vi "Test Sequencer.vi"(7 "Initial Data":T3={"Model Name"=enum."W 501 FLH Std.", "ID"="ID", "Shift"=""}, 8 "Error In":errorcluster, 9 "Initialize":bool, 10 "Inputs":T6) -> (0 "Error Out":errorcluster, 1 "Completed?":bool, 2 "Results":T4, 3 "Results Cluster out":T1, 4 "Graph":dbl[][](array[numeric]), 5 "TS Status":cluster{"Status":string, "Elapsed Time":dbl})   [LabVIEW 2017]
uses:
  controls/All Inputs.ctl
  controls/SACB DI.ctl
  controls/Test Sequencer.ctl
  controls/AC Results.ctl
  controls/Model Name.ctl
  controls/Results Cluster.ctl
  controls/Result Checker.ctl
  GV/Specs.vi
  support/GV/Towerlight GV.vi
panel:
  out "Current State":T5
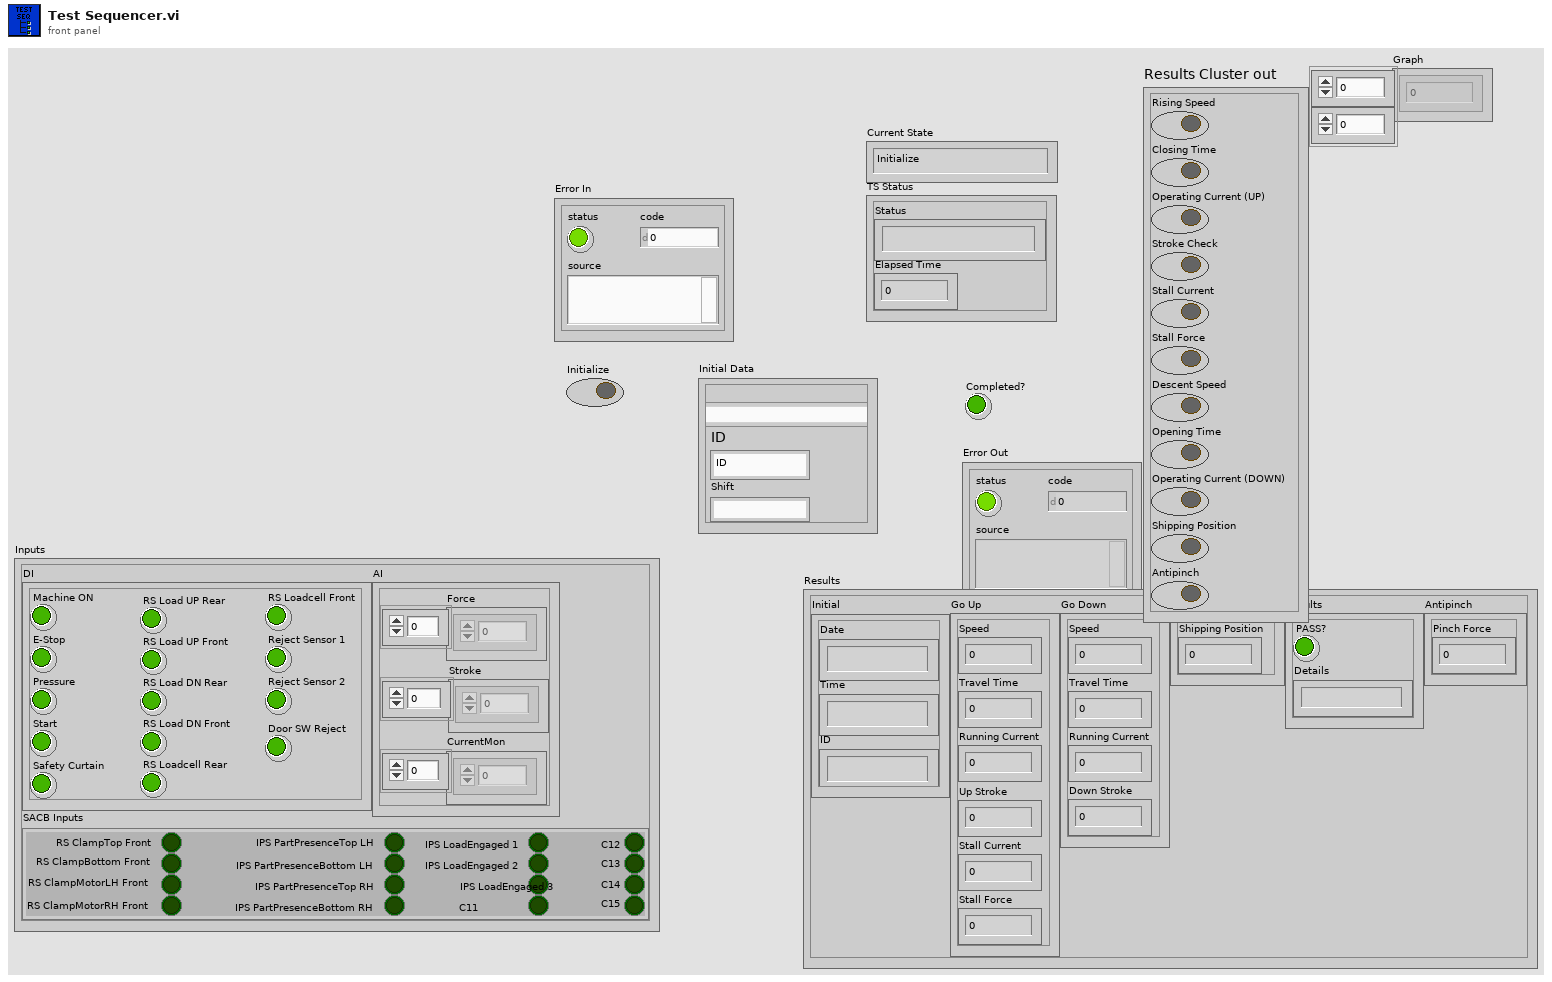
[diagram p1: front panel]
types:
  T1 = typedef "Results Cluster.ctl" = cluster{"Rising Speed":bool, "Closing Time":bool, "Operating Current (UP)":bool, "Stroke Check":bool, "Stall Current":bool, "Stall Force":bool, "Descent Speed":bool, "Opening Time":bool, "Operating Current (DOWN)":bool, "Shipping Position":bool, "Antipinch":bool}
  T2 = typedef "Model Name.ctl" = enum16{"W 501 FLH Std.", "W 501 FRH Std.", "W 601 FR RH Std", "W 601 FR LH Std", "W 601 RR RH Std", "W 601 RR LH Std", "W 601 FR RH AP", "W 601 FR LH AP", "W 601 RR RH AP", "W 601 RR LH AP"}
  T3 = cluster{"Model Name":T2, "ID":string, "Shift":string}
  T4 = typedef "AC Results.ctl" = cluster{"Initial":cluster{"Date":string, "Time":string, "ID":string}, "Go Up":cluster{"Speed":dbl, "Travel Time":dbl, "Running Current":dbl, "Up Stroke":dbl, "Stall Current":dbl, "Stall Force":dbl}, "Go Down":cluster{"Speed":dbl, "Travel Time":dbl, "Running Current":dbl, "Down Stroke":dbl}, "Shipping Position":cluster{"Shipping Position":dbl}, "Results":cluster{"PASS?":bool, "Details":string}, "Antipinch":cluster{"Pinch Force":dbl}}
  T5 = typedef "Test Sequencer.ctl" = enum16{"Initialize", "Clamp", "Homing (DOWN)", "Go UP (Initialization)", "Go Up", "Go DOWN", "Go UP (Loaded)", "Stall Force", "Go DOWN (Loaded)", "Antipinch", "De Initialization", "BSL Flash", "Shipping Position", "De-Clamp", "Result Checker"}
  T6 = typedef "All Inputs.ctl" = cluster{"DI":cluster{"Machine ON":bool, "E-Stop":bool, "Pressure":bool, "Start":bool, "Safety Curtain":bool, "RS Load UP Rear":bool, "RS Load UP Front":bool, "RS Load DN Rear":bool, "RS Load DN Front":bool, "RS Loadcell Rear":bool, "RS Loadcell Front":bool, "Reject Sensor 1":bool, "Reject Sensor 2":bool, "Door SW Reject":bool}, "AI":cluster{"Force":dbl[], "Stroke":dbl[], "CurrentMon":dbl[]}, "SACB Inputs":T7}
  T7 = typedef "SACB DI.ctl" = cluster{"RS ClampTop Front":bool, "RS ClampBottom Front":bool, "RS ClampMotorLH Front":bool, "RS ClampMotorRH Front":bool, "IPS PartPresenceTop LH":bool, "IPS PartPresenceBottom LH":bool, "IPS PartPresenceTop RH":bool, "IPS PartPresenceBottom RH":bool, "IPS LoadEngaged 1":bool, "IPS LoadEngaged 2":bool, "IPS LoadEngaged 3":bool, "C11":bool, "C12":bool, "C13":bool, "C14":bool, "C15":bool}
  T8 = typedef "Result Checker.ctl" = enum16{"Go Up", "Go Down", "Stall Force", "Shipping Position", "Antipinch"}
  T9 = cluster{"Speed":dbl, "Travel Time":dbl, "Running Current":dbl, "Up Stroke":dbl, "Stall Current":dbl, "Stall Force":dbl}
  T10 = cluster{"Speed":dbl, "Travel Time":dbl, "Running Current":dbl, "Down Stroke":dbl}
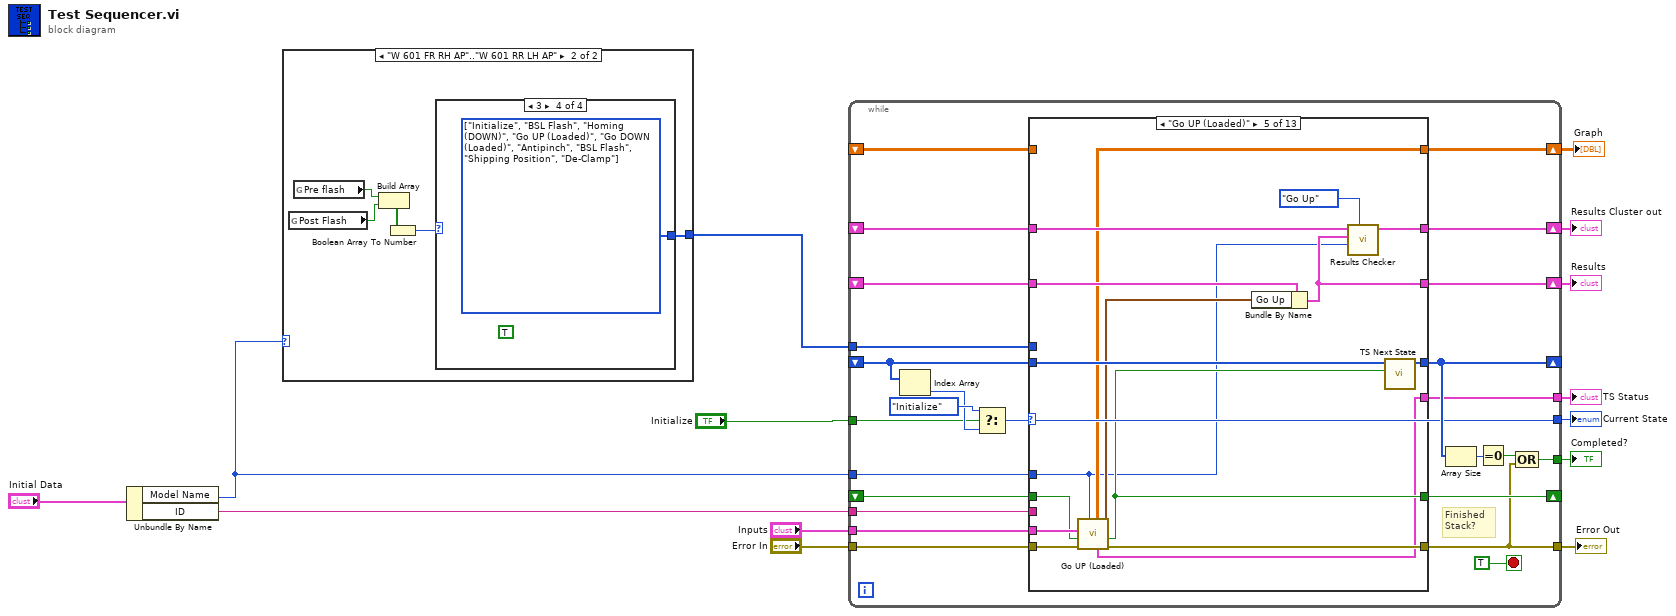
[diagram p0: block diagram]
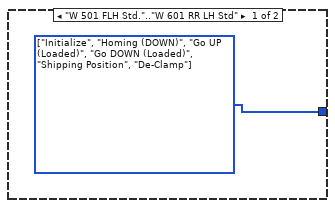
[diagram p2: hidden frame]
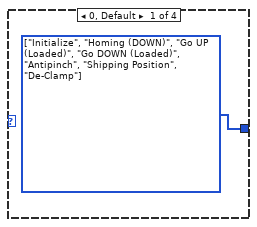
[diagram p3: hidden frame]
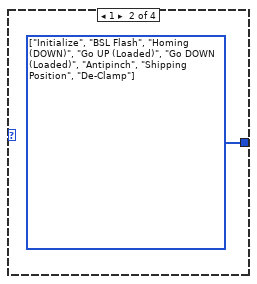
[diagram p4: hidden frame]
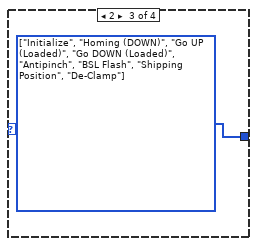
[diagram p5: hidden frame]
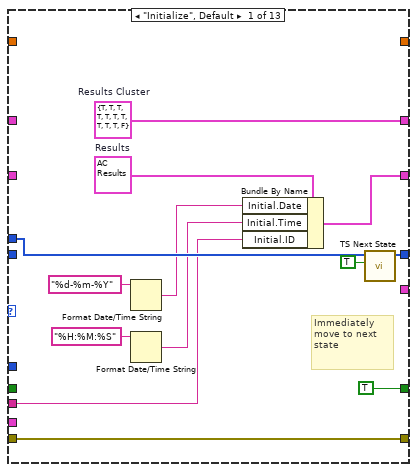
[diagram p6: hidden frame]
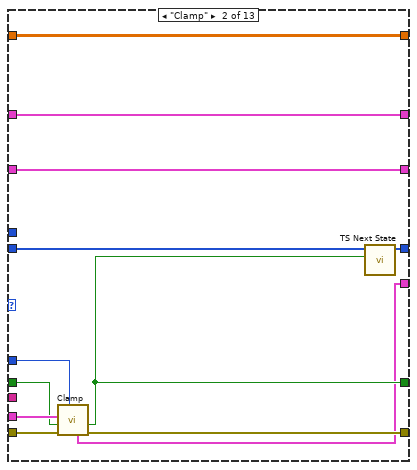
[diagram p7: hidden frame]
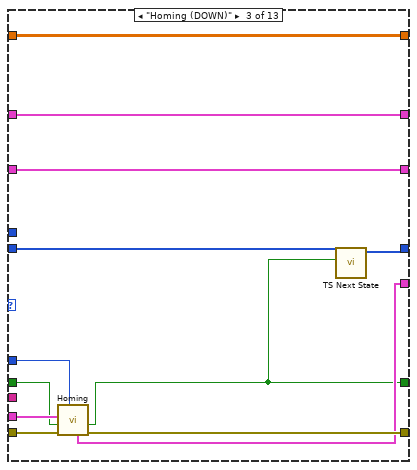
[diagram p8: hidden frame]
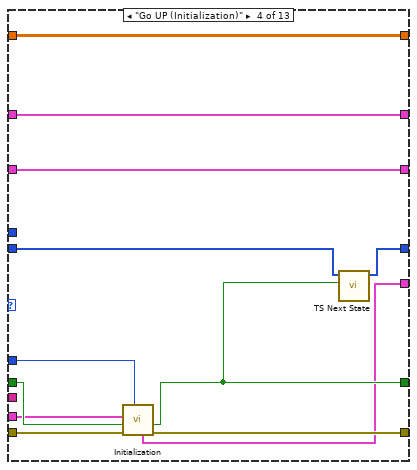
[diagram p9: hidden frame]
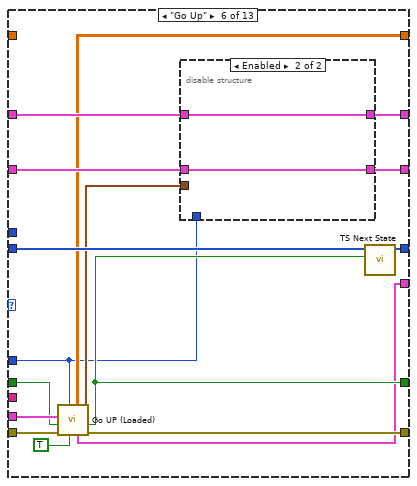
[diagram p10: hidden frame]
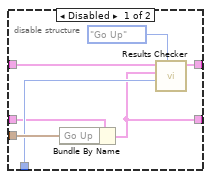
[diagram p11: hidden frame]
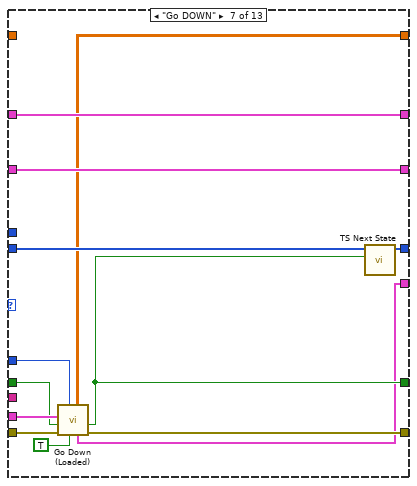
[diagram p12: hidden frame]
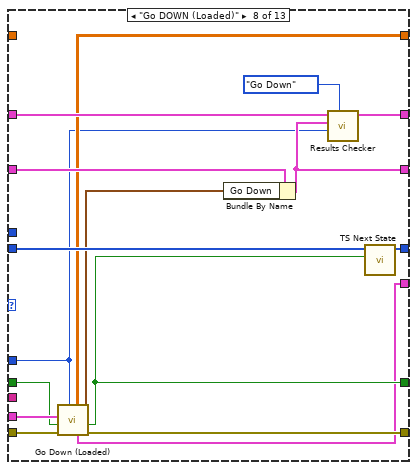
[diagram p13: hidden frame]
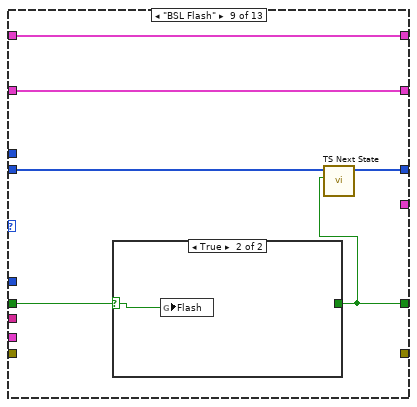
[diagram p14: hidden frame]
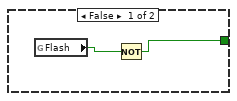
[diagram p15: hidden frame]
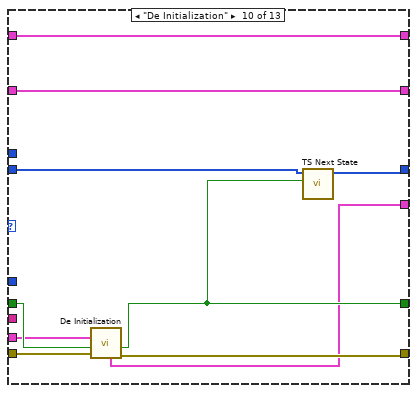
[diagram p16: hidden frame]
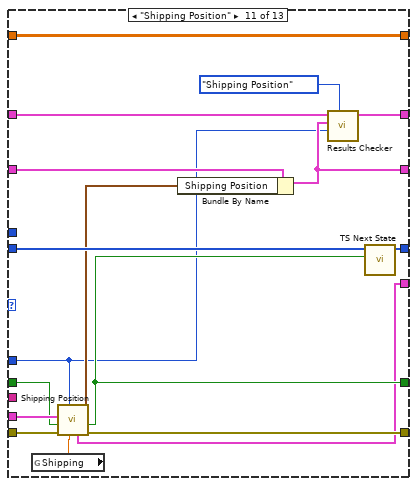
[diagram p17: hidden frame]
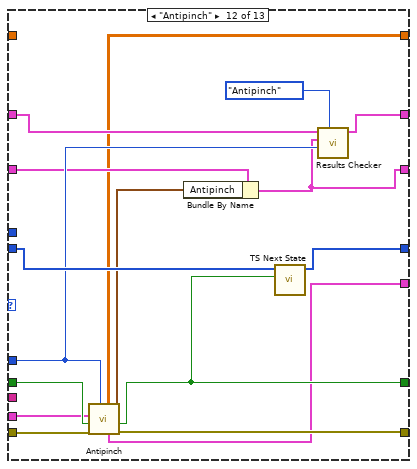
[diagram p18: hidden frame]
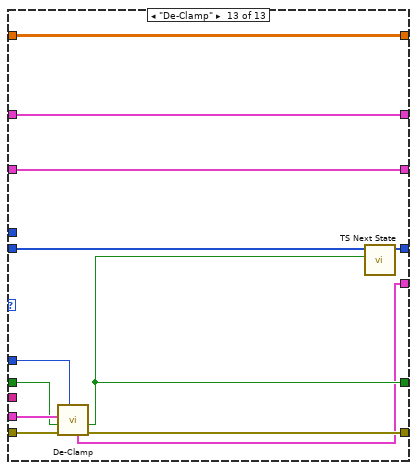
[diagram p19: hidden frame]
diagram:
  n1 = Unbundle By Name("Initial Data") -> ("Model Name"=w2:T2, "ID"=w5:string)
  n2 = case shown="\"W 601 FR RH AP\"..\"W 601 RR LH AP\"" w2 {
    tunnel: [w15 w16] -> w1
    frame "W 501 FLH Std.".."W 601 RR LH Std" {
      w15 = T5[] [enum."Initialize", enum."Homing (DOWN)", enum."Go UP (Loaded)", enum."Go DOWN (Loaded)", enum."Shipping Position", enum."De-Clamp"] items=["Initialize", "Clamp", "Homing (DOWN)", "Go UP (Initialization)", "Go Up", "Go DOWN", "Go UP (Loaded)", "Stall Force", "Go DOWN (Loaded)", "Antipinch", "De Initialization", "BSL Flash", "Shipping Position", "De-Clamp", "Result Checker"]
    }
    frame "W 601 FR RH AP".."W 601 RR LH AP" {
      (unwired) TRUE
      n3 = global read "Specs.vi" "Post Flash"() -> (w19:bool)
      n4 = global read "Specs.vi" "Pre flash"() -> (w20:bool)
      n5 = Build Array(w20, w19) -> (w17:bool[])
      n6 = Boolean Array To Number(Boolean array=w17) -> (number=w18:u32)
      n7 = case shown="3" w18 {
        tunnel: [w21 w22 w23 w24] -> w16
        frame 0, Default {
          w21 = T5[] [enum."Initialize", enum."Homing (DOWN)", enum."Go UP (Loaded)", enum."Go DOWN (Loaded)", enum."Antipinch", enum."Shipping Position", enum."De-Clamp"] items=["Initialize", "Clamp", "Homing (DOWN)", "Go UP (Initialization)", "Go Up", "Go DOWN", "Go UP (Loaded)", "Stall Force", "Go DOWN (Loaded)", "Antipinch", "De Initialization", "BSL Flash", "Shipping Position", "De-Clamp", "Result Checker"]
        }
        frame 1 {
          w22 = T5[] [enum."Initialize", enum."BSL Flash", enum."Homing (DOWN)", enum."Go UP (Loaded)", enum."Go DOWN (Loaded)", enum."Antipinch", enum."Shipping Position", enum."De-Clamp"] items=["Initialize", "Clamp", "Homing (DOWN)", "Go UP (Initialization)", "Go Up", "Go DOWN", "Go UP (Loaded)", "Stall Force", "Go DOWN (Loaded)", "Antipinch", "De Initialization", "BSL Flash", "Shipping Position", "De-Clamp", "Result Checker"]
        }
        frame 2 {
          w23 = T5[] [enum."Initialize", enum."Homing (DOWN)", enum."Go UP (Loaded)", enum."Go DOWN (Loaded)", enum."Antipinch", enum."BSL Flash", enum."Shipping Position", enum."De-Clamp"] items=["Initialize", "Clamp", "Homing (DOWN)", "Go UP (Initialization)", "Go Up", "Go DOWN", "Go UP (Loaded)", "Stall Force", "Go DOWN (Loaded)", "Antipinch", "De Initialization", "BSL Flash", "Shipping Position", "De-Clamp", "Result Checker"]
        }
        frame 3 {
          w24 = T5[] [enum."Initialize", enum."BSL Flash", enum."Homing (DOWN)", enum."Go UP (Loaded)", enum."Go DOWN (Loaded)", enum."Antipinch", enum."BSL Flash", enum."Shipping Position", enum."De-Clamp"] items=["Initialize", "Clamp", "Homing (DOWN)", "Go UP (Initialization)", "Go Up", "Go DOWN", "Go UP (Loaded)", "Stall Force", "Go DOWN (Loaded)", "Antipinch", "De Initialization", "BSL Flash", "Shipping Position", "De-Clamp", "Result Checker"]
        }
      }
    }
  }
  n8 = while {
    tunnel: w1 -> [w49]
    shift-right: [w40] -> _
    shift-left: _ -> [w48]
    tunnel: "Initialize" -> [w36]
    shift-right: [w44] -> _
    shift-left: _ -> [w43]
    tunnel: "Error In" -> [w42]
    tunnel: [w37] -> w12
    tunnel: "Inputs" -> [w41]
    tunnel: [w35] -> w10
    tunnel: w2 -> [w34]
    tunnel: [w33] -> w9
    tunnel: w5 -> [w32]
    shift-right: [w31] -> w7
    shift-left: _ -> [w30]
    tunnel: [w29] -> w8
    shift-right: [w28] -> w4
    shift-left: _ -> [w27]
    shift-right: [w26] -> w3
    shift-left: _ -> [w25]
    stop <- TRUE stop-if-true
    # "Finished Stack?"
    n9 = Index Array(array=w48) -> (element=w46:T5)  [unwired: 1 in]
    n10 = Select(t=Test_Sequencer."Initialize", s=w36, f=w46) -> (s? t:f=w33:T5)
    n11 = case shown="\"Go UP (Loaded)\"" w33 {
      tunnel: w49 -> [w60 _ _ _ _ _ _ _ _ _ _ _ _]
      tunnel: [w62 w74 w77 w91 w114 w130 w152 w168 w173 w182 w204 w214 w232] -> w40
      tunnel: w48 -> [_ w73 w79 w92 w113 w129 w151 w167 w172 w183 w203 w215 w231]
      tunnel: [TRUE w68 w78 w93 w108 w124 w146 w162 w171 w181 w198 w216 w226] -> w44
      tunnel: w43 -> [_ w69 w83 w97 w109 w125 w147 w163 w174 w185 w199 w218 w227]
      tunnel: w42 -> [w58 w72 w86 w98 w112 w128 w150 w166 _ w187 w202 w220 w230]
      tunnel: [w58 w71 w85 w94 w111 w127 w149 w165 _ w186 w201 w219 w229] -> w37
      tunnel: w41 -> [_ w70 w84 w96 w110 w126 w148 w164 _ w184 w200 w217 w228]
      tunnel: w34 -> [_ w64 w75 w95 w99 w115 w140 w153 _ _ w188 w211 w222]
      tunnel: w32 -> [w51 _ _ _ _ _ _ _ _ _ _ _ _]
      tunnel: [w55 w67 w82 w88 w104 w120 w143 w155 w169 w178 w194 w206 w225] -> w31
      tunnel: w30 -> [_ w67 w82 w88 w105 w121 w143 w160 w169 w178 w195 w208 w225]
      tunnel: [_ w66 w81 w90 w107 w123 w145 w161 _ w180 w197 w213 w224] -> w29
      tunnel: [w50 w65 w80 w89 w103 w119 w144 w157 w170 w179 w193 w209 w223] -> w28
      tunnel: w27 -> [_ w65 w80 w89 w102 w118 w144 w156 w170 w179 w192 w212 w223]
      tunnel: [_ w63 w76 w87 w100 w116 w142 w154 _ _ w190 w205 w221] -> w26
      tunnel: w25 -> [_ w63 w76 w87 _ _ _ _ _ _ w190 _ w221]
      frame "Initialize", Default {
        w50 = T1 {"Rising Speed"=TRUE, "Closing Time"=TRUE, "Operating Current (UP)"=TRUE, "Stroke Check"=TRUE, "Stall Current"=TRUE, "Stall Force"=TRUE, "Descent Speed"=TRUE, "Opening Time"=TRUE, "Operating Current (DOWN)"=TRUE, "Shipping Position"=TRUE, "Antipinch"=FALSE}  # Results Cluster
        w56 = T4 {"Initial"={"Date"="", "Time"="", "ID"=""}, "Go Up"={"Speed"=0.0, "Travel Time"=0.0, "Running Current"=0.0, "Up Stroke"=0.0, "Stall Current"=0.0, "Stall Force"=0.0}, "Go Down"={"Speed"=0.0, "Travel Time"=0.0, "Running Current"=0.0, "Down Stroke"=0.0}, "Shipping Position"={"Shipping Position"=0.0}, "Results"={"PASS?"=FALSE, "Details"=""}, "Antipinch"={"Pinch Force"=0.0}}  # Results
        # "Immediately move to next state"
        n12 = Format Date/Time String(time format string (%c)="%d-%m-%Y") -> (date/time string=w53:string)  [unwired: 2 in]
        n13 = Format Date/Time String(time format string (%c)="%H:%M:%S") -> (date/time string=w52:string)  [unwired: 2 in]
        n14 = Bundle By Name(cluster=w56, "Initial.Date"=w53, "Initial.Time"=w52, "Initial.ID"=w51) -> (w55:T4)
        n15 = call "TS Next State.vi"("Next State?"=TRUE, "Array in"=w60) -> ("Array out"=w62:T5[])  [unwired: 9 in]
      }
      frame "Clamp" {
        n16 = call "Clamp.vi"("Model Name"=w64, "Error In"=w72, "Intialize?"=w69, "Inputs"=w70) -> ("error out"=w71:errorcluster, "Completed"=w68:bool, "Status"=w66:cluster{"Status":string, "Elapsed Time":dbl})  [unwired: 5 in]
        n17 = call "TS Next State.vi"("Next State?"=w68, "Array in"=w73) -> ("Array out"=w74:T5[])  [unwired: 9 in]
      }
      frame "Homing (DOWN)" {
        n18 = call "Homing.vi"("Model Name"=w75, "Error In"=w86, "Intialize?"=w83, "Inputs"=w84) -> ("error out"=w85:errorcluster, "Completed"=w78:bool, "Status"=w81:cluster{"Status":string, "Elapsed Time":dbl})  [unwired: 5 in]
        n19 = call "TS Next State.vi"("Next State?"=w78, "Array in"=w79) -> ("Array out"=w77:T5[])  [unwired: 9 in]
      }
      frame "Go UP (Initialization)" {
        n20 = call "Initialization.vi"("Model Name"=w95, "Error In"=w98, "Intialize?"=w97, "Inputs"=w96) -> ("error out"=w94:errorcluster, "Completed"=w93:bool, "Status"=w90:cluster{"Status":string, "Elapsed Time":dbl})  [unwired: 4 in, 1 out]
        n21 = call "TS Next State.vi"("Next State?"=w93, "Array in"=w92) -> ("Array out"=w91:T5[])  [unwired: 9 in]
      }
      frame "Go UP (Loaded)" {
        n22 = call "Go UP (Loaded).vi"("Model Name"=w99, "Error In"=w112, "Intialize?"=w109, "Inputs"=w110) -> ("error out"=w111:errorcluster, "Completed"=w108:bool, "Results"=w106:T9, "Status"=w107:cluster{"Status":string, "Elapsed Time":dbl}, "Graph"=w100:dbl[][])  [unwired: 3 in]
        n23 = Bundle By Name(cluster=w105, "Go Up"=w106) -> (w104:T4)
        n24 = call "Results Checker.vi"("Test Name"=Result_Checker."Go Up", "Model Name"=w99, "Results"=w104, "Results Cluster"=w102) -> ("Results Cluster out"=w103:T1)  [unwired: 7 in]
        n25 = call "TS Next State.vi"("Next State?"=w108, "Array in"=w113) -> ("Array out"=w114:T5[])  [unwired: 9 in]
      }
      frame "Go Up" {
        n26 = call "Go UP (Loaded).vi"("Skip Loading?"=TRUE, "Model Name"=w115, "Error In"=w128, "Intialize?"=w125, "Inputs"=w126) -> ("error out"=w127:errorcluster, "Completed"=w124:bool, "Results"=w122:T9, "Status"=w123:cluster{"Status":string, "Elapsed Time":dbl}, "Graph"=w116:dbl[][])  [unwired: 2 in]
        n27 = disable-structure shown="Enabled" {
          disable-tunnel: w122 -> [w137 _]
          disable-tunnel: w115 -> [w136 _]
          disable-tunnel: w121 -> [w135 w138]
          disable-tunnel: [w134 w138] -> w120
          disable-tunnel: [w133 w139] -> w119
          disable-tunnel: w118 -> [w132 w139]
          frame Disabled {
            n28 = Bundle By Name(cluster=w135, "Go Up"=w137) -> (w134:T4)
            n29 = call "Results Checker.vi"("Test Name"=Result_Checker."Go Up", "Model Name"=w136, "Results"=w134, "Results Cluster"=w132) -> ("Results Cluster out"=w133:T1)  [unwired: 7 in]
          }
          frame Enabled {
          }
        }
        n30 = call "TS Next State.vi"("Next State?"=w124, "Array in"=w129) -> ("Array out"=w130:T5[])  [unwired: 9 in]
      }
      frame "Go DOWN" {
        n31 = call "Go Down (Loaded).vi"("Skip Load?"=TRUE, "Model Name"=w140, "Error In"=w150, "Intialize?"=w147, "Inputs"=w148) -> ("error out"=w149:errorcluster, "Completed"=w146:bool, "Status"=w145:cluster{"Status":string, "Elapsed Time":dbl}, "Array"=w142:dbl[][])  [unwired: 2 in, 1 out]
        n32 = call "TS Next State.vi"("Next State?"=w146, "Array in"=w151) -> ("Array out"=w152:T5[])  [unwired: 9 in]
      }
      frame "Go DOWN (Loaded)" {
        n33 = call "Go Down (Loaded).vi"("Model Name"=w153, "Error In"=w166, "Intialize?"=w163, "Inputs"=w164) -> ("error out"=w165:errorcluster, "Completed"=w162:bool, "Results"=w159:T10, "Status"=w161:cluster{"Status":string, "Elapsed Time":dbl}, "Array"=w154:dbl[][])  [unwired: 3 in]
        n34 = Bundle By Name(cluster=w160, "Go Down"=w159) -> (w155:T4)
        n35 = call "Results Checker.vi"("Test Name"=Result_Checker."Go Down", "Model Name"=w153, "Results"=w155, "Results Cluster"=w156) -> ("Results Cluster out"=w157:T1)  [unwired: 7 in]
        n36 = call "TS Next State.vi"("Next State?"=w162, "Array in"=w167) -> ("Array out"=w168:T5[])  [unwired: 9 in]
      }
      frame "BSL Flash" {
        n37 = case shown="True" w174 {
          selector: w174 -> [_ w177]
          tunnel: [w175 _] -> w171
          frame False {
            n38 = global read "Towerlight GV.vi" "Flash"() -> (w176:bool)
            n39 = Not(x=w176) -> (.not. x?=w175:bool)
          }
          frame True {
            n40 = global write "Towerlight GV.vi" "Flash"(w177) -> ()
          }
        }
        n41 = call "TS Next State.vi"("Next State?"=w171, "Array in"=w172) -> ("Array out"=w173:T5[])  [unwired: 9 in]
      }
      frame "De Initialization" {
        n42 = call "De Initialization.vi"("Error In"=w187, "Intialize?"=w185, "Inputs"=w184) -> ("error out"=w186:errorcluster, "Completed"=w181:bool, "Status"=w180:cluster{"Status":string, "Elapsed Time":dbl})  [unwired: 4 in, 2 out]
        n43 = call "TS Next State.vi"("Next State?"=w181, "Array in"=w183) -> ("Array out"=w182:T5[])  [unwired: 9 in]
      }
      frame "Shipping Position" {
        n44 = global read "Specs.vi" "Shipping"() -> (w189:dbl)
        n45 = call "Shipping Position.vi"("Shipping"=w189, "Model Name"=w188, "Error In"=w202, "Intialize?"=w199, "Inputs"=w200) -> ("error out"=w201:errorcluster, "Completed"=w198:bool, "Results"=w196:cluster{"Shipping Position":dbl}, "Status"=w197:cluster{"Status":string, "Elapsed Time":dbl})  [unwired: 3 in]
        n46 = Bundle By Name(cluster=w195, "Shipping Position"=w196) -> (w194:T4)
        n47 = call "Results Checker.vi"("Test Name"=Result_Checker."Shipping Position", "Model Name"=w188, "Results"=w194, "Results Cluster"=w192) -> ("Results Cluster out"=w193:T1)  [unwired: 7 in]
        n48 = call "TS Next State.vi"("Next State?"=w198, "Array in"=w203) -> ("Array out"=w204:T5[])  [unwired: 9 in]
      }
      frame "Antipinch" {
        n49 = call "Antipinch.vi"("Model Name"=w211, "Error In"=w220, "Intialize?"=w218, "Inputs"=w217) -> ("error out"=w219:errorcluster, "Completed"=w216:bool, "Results"=w207:cluster{"Pinch Force":dbl}, "Status"=w213:cluster{"Status":string, "Elapsed Time":dbl}, "Graph"=w205:dbl[][])  [unwired: 3 in]
        n50 = Bundle By Name(cluster=w208, "Antipinch"=w207) -> (w206:T4)
        n51 = call "TS Next State.vi"("Next State?"=w216, "Array in"=w215) -> ("Array out"=w214:T5[])  [unwired: 9 in]
        n52 = call "Results Checker.vi"("Test Name"=Result_Checker."Antipinch", "Model Name"=w211, "Results"=w206, "Results Cluster"=w212) -> ("Results Cluster out"=w209:T1)  [unwired: 7 in]
      }
      frame "De-Clamp" {
        n53 = call "De-Clamp.vi"("Model Name"=w222, "Error In"=w230, "Intialize?"=w227, "Inputs"=w228) -> ("error out"=w229:errorcluster, "Completed"=w226:bool, "Status"=w224:cluster{"Status":string, "Elapsed Time":dbl})  [unwired: 5 in]
        n54 = call "TS Next State.vi"("Next State?"=w226, "Array in"=w231) -> ("Array out"=w232:T5[])  [unwired: 9 in]
      }
    }
    n55 = Array Size(array=w40) -> (size(s)=w39:i32)
    n56 = Equal To 0?(x=w39) -> (x = 0?=w38:bool)
    n57 = Compound Arithmetic op=OR(w38, w37) -> (w35:bool)
  }
  "Error Out" <- w12
  "Completed?" <- w10
  "Current State" <- w9
  "TS Status" <- w8
  "Results" <- w7
  "Results Cluster out" <- w4
  "Graph" <- w3
